vi "Read IK Recording Error File Write Cells.vi"(5 "Reason Column Letter":string="D", 7 "Depth Column Letter":string="C", 8 "error in (no error)":errorcluster, 9 "Row Offset In":i32, 10 "IK Recording Data file":path, 11 "NI_report in":refnum<class "NI_report.lvclass">) -> (0 "error out":errorcluster, 1 "all rows":string[][](array[string]), 2 "Row Offset Out":i32, 3 "NI_report out":refnum<class "NI_report.lvclass">)   [LabVIEW 2016]
uses:
  <vilib>/Utility/NIReport.llb/NI_report.lvclass
  <vilib>/Utility/file.llb/Read Delimited Spreadsheet (string).vi
panel:
  out "subarray":string[][](array[string])
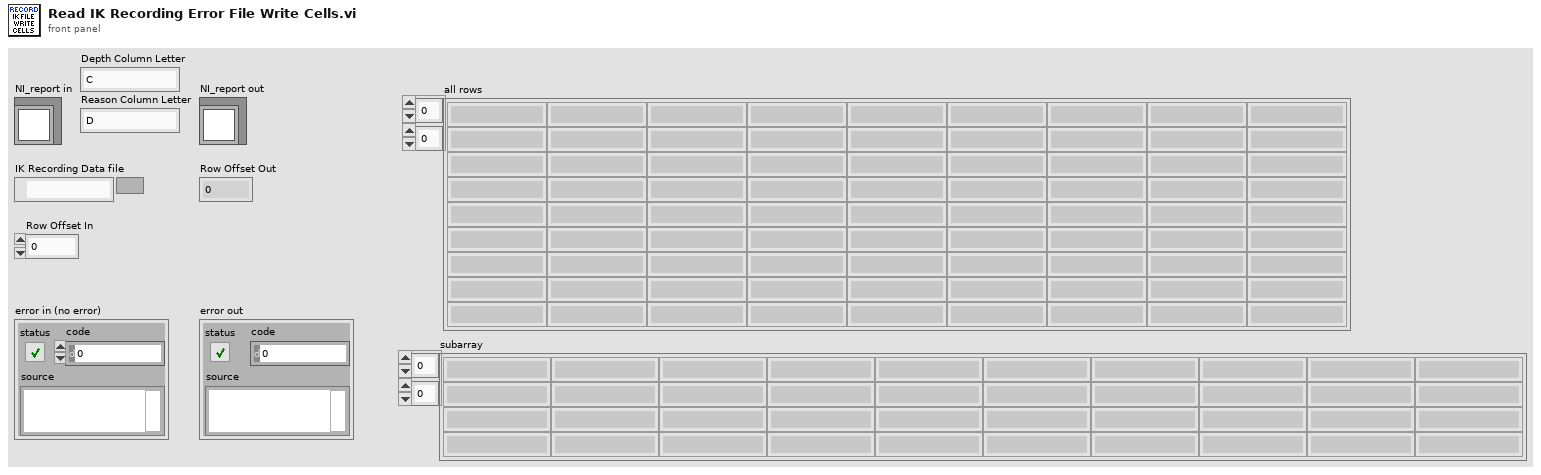
[diagram p1: front panel]
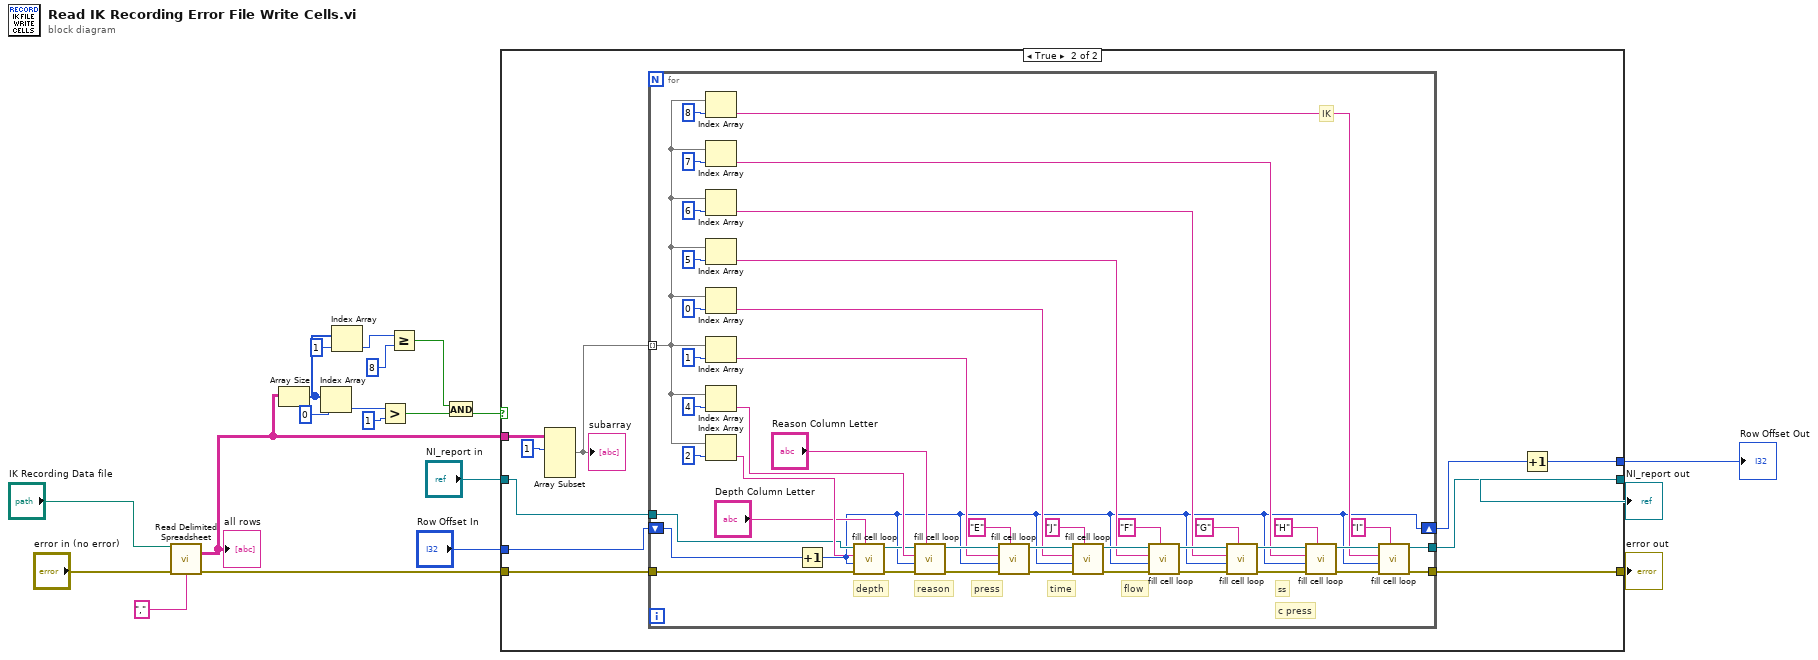
[diagram p0: block diagram]
diagram:
  n1 = call-poly <vilib>:"Read Delimited Spreadsheet.vi"("file path (dialog if empty)"="IK Recording Data file", "error in (no error)"="error in (no error)", "delimiter (\\t)"="," ("delimiter (\\t)")) -> ("all rows"=w11:string[][], "error out"=w20:errorcluster)  [unwired: 7 in, 4 out]
  "all rows" <- w11
  n2 = Array Size(array=w11) -> (size(s)=w5:i32[])
  n3 = Index Array(array=w5, index=0) -> (element=w10:i32)
  n4 = Index Array(array=w5, index=1) -> (element=w3:i32)
  n5 = Greater?(x=w10, y=1) -> (0:w8:bool)
  n6 = Greater Or Equal?(x=w3, y=8) -> (x >= y?=w1:bool)
  n7 = And(x=w1, y=w8) -> (x .and. y?=w7:bool)
  n8 = case shown="True" w7 {
    tunnel: w20 -> [w21 w33]
    tunnel: [w21 w32] -> w18
    tunnel: [w23 w31] -> w17
    tunnel: [w22 w24] -> w16
    tunnel: "NI_report in" -> [w23 w29]
    tunnel: "Row Offset In" -> [w22 w28]
    tunnel: w11 -> [_ w25]
    frame False {
    }
    frame True {
      n9 = Array Subset(array=w25, index (row)=1 ("index")) -> (w27:string[][])  [unwired: 3 in]
      "subarray" <- w27
      n10 = for {
        tunnel: w27 -> [w40] mode=indexing
        shift-right: [w35] -> w30
        shift-left: w28 -> [w78]
        tunnel: w29 -> [w70]
        tunnel: w33 -> [w73]
        tunnel: [w36] -> w32
        tunnel: [w37] -> w31
        # "IK"
        # "ss"
        # "c press"
        # "flow"
        # "time"
        # "press"
        # "reason"
        # "depth"
        n11 = Index Array(array=w40, index=8) -> (element=w38:string)
        n12 = Index Array(array=w40, index=7) -> (element=w42:string)
        n13 = Index Array(array=w40, index=6) -> (element=w49:string)
        n14 = Index Array(array=w40, index=5) -> (element=w52:string)
        n15 = Index Array(array=w40, index=0) -> (element=w53:string)
        n16 = Index Array(array=w40, index=1) -> (element=w54:string)
        n17 = Index Array(array=w40, index=4) -> (element=w74:string)
        n18 = Index Array(array=w40, index=2) -> (element=w71:string)
        n19 = Increment(x=w78) -> (x+1=w35:i32)
        n20 = call "fill cell loop.vi"("Column Letter"="Depth Column Letter", "error in (no error)"=w73, "Row"=w35, "String"=w71, "NI_report in"=w70) -> ("error out"=w72:errorcluster, "NI_report out"=w69:refnum<class "NI_report.lvclass">)  [unwired: 5 in]
        n21 = call "fill cell loop.vi"("Column Letter"="Reason Column Letter", "error in (no error)"=w72, "Row"=w35, "String"=w74, "NI_report in"=w69) -> ("error out"=w64:errorcluster, "NI_report out"=w65:refnum<class "NI_report.lvclass">)  [unwired: 5 in]
        n22 = call "fill cell loop.vi"("Column Letter"="E" ("String"), "error in (no error)"=w64, "Row"=w35, "String"=w54, "NI_report in"=w65) -> ("error out"=w67:errorcluster, "NI_report out"=w66:refnum<class "NI_report.lvclass">)  [unwired: 5 in]
        n23 = call "fill cell loop.vi"("Column Letter"="J", "error in (no error)"=w67, "Row"=w35, "String"=w53, "NI_report in"=w66) -> ("error out"=w62:errorcluster, "NI_report out"=w63:refnum<class "NI_report.lvclass">)  [unwired: 5 in]
        n24 = call "fill cell loop.vi"("Column Letter"="F", "error in (no error)"=w62, "Row"=w35, "String"=w52, "NI_report in"=w63) -> ("error out"=w60:errorcluster, "NI_report out"=w61:refnum<class "NI_report.lvclass">)  [unwired: 5 in]
        n25 = call "fill cell loop.vi"("Column Letter"="G", "error in (no error)"=w60, "Row"=w35, "String"=w49, "NI_report in"=w61) -> ("error out"=w48:errorcluster, "NI_report out"=w47:refnum<class "NI_report.lvclass">)  [unwired: 5 in]
        n26 = call "fill cell loop.vi"("Column Letter"="H", "error in (no error)"=w48, "Row"=w35, "String"=w42, "NI_report in"=w47) -> ("error out"=w46:errorcluster, "NI_report out"=w45:refnum<class "NI_report.lvclass">)  [unwired: 5 in]
        n27 = call "fill cell loop.vi"("Column Letter"="I", "error in (no error)"=w46, "Row"=w35, "String"=w38, "NI_report in"=w45) -> ("error out"=w36:errorcluster, "NI_report out"=w37:refnum<class "NI_report.lvclass">)  [unwired: 5 in]
      }
      n28 = Increment(x=w30) -> (x+1=w24:i32)
    }
  }
  "error out" <- w18
  "NI_report out" <- w17
  "Row Offset Out" <- w16
